vi "JK触发器逻辑功能的测试.vi"(0 "J":bool, 1 "R":bool, 2 "cp":bool, 3 "K":bool, 4 "S":bool) -> (6 "Q":bool, 7 "Q`":bool)   [LabVIEW 2018]
panel:
  in  "结束":bool
  # "下降沿触发的JK触发器"
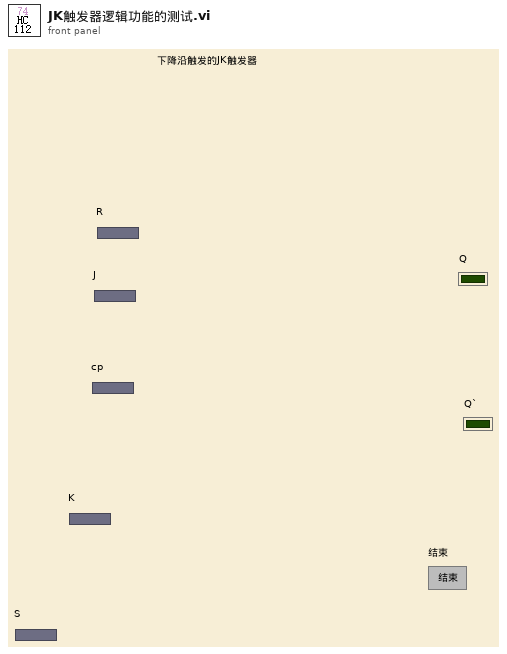
[diagram p1: front panel]
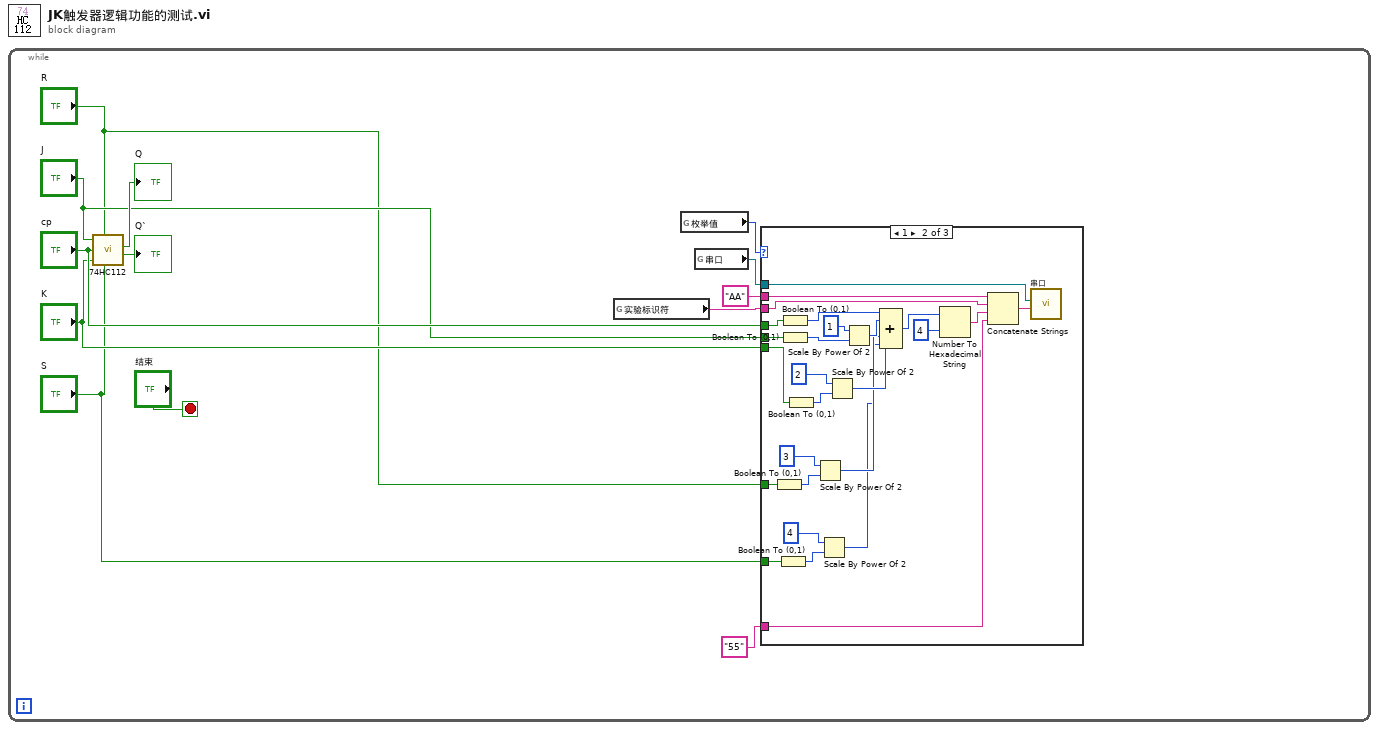
[diagram p0: block diagram]
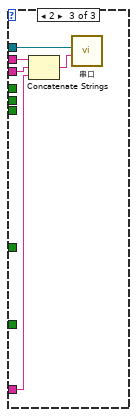
[diagram p3: hidden frame]
diagram:
  n1 = while {
    stop <- "结束" stop-if-true
    n2 = call "74HC112.vi"("J"="J", "R"="R", "cp"="cp", "K"="K", "S"="S") -> ("Q"=→"Q":bool, "Q`"=→"Q`":bool)  [unwired: 2 in]
    n3 = global read "全局变量.vi" "实验标识符"() -> (w8:string)
    n4 = global read "全局变量.vi" "枚举值"() -> (w10:i8)
    n5 = global read "全局变量.vi" "串口"() -> (w9:refnum<visa-resource-name>)
    n6 = case shown="1" w10 {
      tunnel: w9 -> [_ w34 w42]
      tunnel: w8 -> [_ w33 w43]
      tunnel: "55" -> [_ w32 w40]
      tunnel: "AA" -> [_ w31 w41]
      tunnel: "cp" -> [_ w18 _]
      tunnel: "J" -> [_ w17 _]
      tunnel: "K" -> [_ w16 _]
      tunnel: "R" -> [_ w15 _]
      tunnel: "S" -> [_ w14 _]
      frame 0, Default {
      }
      frame 1 {
        n7 = Boolean To (0,1)(Boolean=w15) -> (0, 1=w24:i16)
        n8 = Boolean To (0,1)(Boolean=w14) -> (0, 1=w21:i16)
        n9 = Boolean To (0,1)(Boolean=w18) -> (0, 1=w38:i16)
        n10 = Boolean To (0,1)(Boolean=w17) -> (0, 1=w36:i16)
        n11 = Boolean To (0,1)(Boolean=w16) -> (0, 1=w26:i16)
        n12 = Scale By Power Of 2(n=3, x=w24) -> (x*2^n=w22:i16)
        n13 = Scale By Power Of 2(n=4, x=w21) -> (x*2^n=w19:i16)
        n14 = Scale By Power Of 2(n=2, x=w26) -> (x*2^n=w27:i16)
        n15 = Scale By Power Of 2(n=1, x=w36) -> (x*2^n=w37:i16)
        n16 = Compound Arithmetic op=ADD ("复合运算")(w38, w37, w27, w22, w19) -> (w30:i16)
        n17 = Number To Hexadecimal String(1:4, 2:w30) -> (0:w28:string)
        n18 = Concatenate Strings(w31, w33, w28, w32) -> (w39:string)
        n19 = call "串口.vi"("字符串"=w39, "VISA resource name"=w34) -> ()  [unwired: 10 in]
      }
      frame 2 {
        n20 = Concatenate Strings(w41, w43, w40) -> (w44:string)
        n21 = call "串口.vi"("字符串"=w44, "VISA resource name"=w42) -> ()  [unwired: 10 in]
      }
    }
  }
